vi "Create Matrix.vi"(3 "Array":dbl[][](array[numeric])=[[-200.0, -0.1], [-400.0, -0.2], [-600.0, -0.5], [-800.0, -1.0], [-1000.0, -100.0]]) -> (1 "Real Matrix":T1)   [LabVIEW 2015]
uses:
  <vilib>/Analysis/Matrix/Datatypes/RealMatrix.ctl
  <vilib>/Analysis/Matrix/Numeric/Conversions/Array To Matrix - RA2.vi
  <vilib>/Analysis/Matrix/NI_Matrix.lvlib
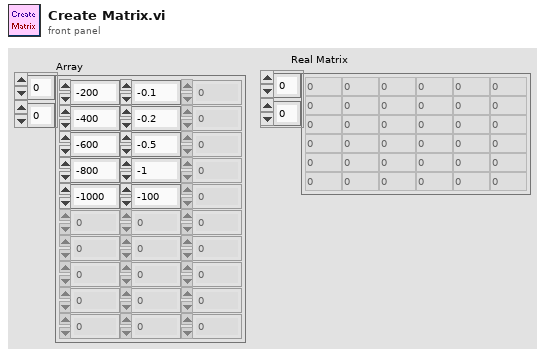
[diagram p1: front panel]
types:
  T1 = typedef "NI_Matrix.lvlib/RealMatrix.ctl" = dbl[][]
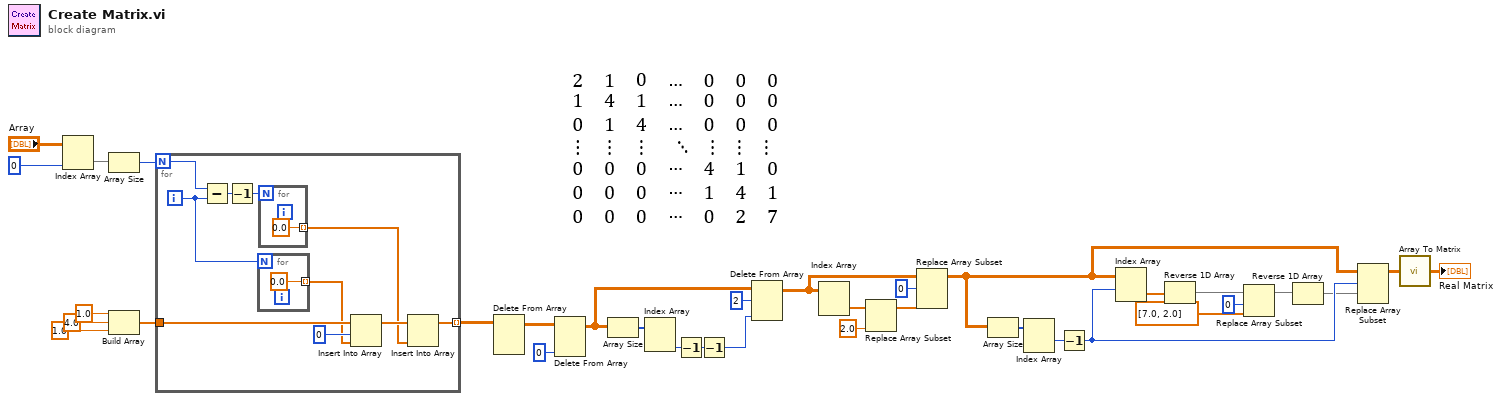
[diagram p0: block diagram]
diagram:
  n1 = Index Array(array="Array", index (col)=0 ("disabled index (col)")) -> (element=w33:dbl[])  [unwired: 1 in]
  n2 = Array Size(array=w33) -> (size(s)=w27:i32)
  n3 = Build Array(1.0, 4.0, 1.0) -> (w28:dbl[])
  n4 = for {
    N: w27 -> [w44]
    tunnel: w28 -> [w42]
    tunnel: [w37] -> w26 mode=indexing
    i -> [w43]
    n5 = Subtract(x=w44, y=w43) -> (x-y=w36:i32)
    n6 = Decrement(x=w36) -> (x-1=w35:i32)
    n7 = for {
      N: w43 -> [_]
      tunnel: [0.0] -> w40 mode=indexing
    }
    n8 = for {
      N: w35 -> [_]
      tunnel: [0.0] -> w38 mode=indexing
    }
    n9 = Insert Into Array(array=w42, index=0, new element=w40) -> (w39:dbl[])
    n10 = Insert Into Array(array=w39, new element=w38) -> (w37:dbl[])  [unwired: 1 in]
  }
  n11 = Delete From Array(array=w26) -> (array with subset deleted=w25:dbl[][])  [unwired: 3 in, 1 out]
  n12 = Delete From Array(array=w25, index (col)=0 ("disabled index (col)")) -> (array with subset deleted=w22:dbl[][])  [unwired: 2 in, 1 out]
  n13 = Array Size(array=w22) -> (size(s)=w23:i32[])
  n14 = Index Array(array=w23) -> (element #2=w21:i32)  [unwired: 2 in, 1 out]
  n15 = Decrement(x=w21) -> (x-1=w19:i32)
  n16 = Decrement(x=w19) -> (x-1=w13:i32)
  n17 = Delete From Array(array=w22, length=2, index (col)=w13) -> (array with subset deleted=w16:dbl[][])  [unwired: 1 in, 1 out]
  n18 = Index Array(array=w16) -> (element=w18:dbl[])  [unwired: 2 in]
  n19 = Replace Array Subset(array=w18, new element=2.0 ("new element/subarray")) -> (w15:dbl[])  [unwired: 1 in]
  n20 = Replace Array Subset(array=w16, new element=w15, index (row)=0) -> (w3:dbl[][])  [unwired: 1 in]
  n21 = Array Size(array=w3) -> (size(s)=w12:i32[])
  n22 = Index Array(array=w12) -> (element #1=w11:i32)  [unwired: 2 in, 1 out]
  n23 = Decrement(x=w11) -> (x-1=w5:i32)
  n24 = Index Array(array=w3, index (row)=w5) -> (element=w10:dbl[])  [unwired: 1 in]
  n25 = Reverse 1D Array(array=w10) -> (reversed array=w8:dbl[])
  n26 = Replace Array Subset(array=w8, new element=dbl[] [7.0, 2.0], index=0 ("index (row)")) -> (w6:dbl[])
  n27 = Reverse 1D Array(array=w6) -> (reversed array=w4:dbl[])
  n28 = Replace Array Subset(array=w3, new element=w4, index (row)=w5) -> (w2:dbl[][])  [unwired: 1 in]
  n29 = call-poly <vilib>:"Array To Matrix.vi"("Real 2D Array"=w2) -> ("Real Matrix"=→"Real Matrix":T1)
